vi "AMZ_S3_APIHLP_Convert MFA Delete String to Enum.vi"(4 "MFA Delete String":string) -> (1 "MFA Delete":T1)   [LabVIEW 2015, in "LV Interface for Amazon S3.lvlib"]
doc: "Convert the Storage Class represented as a String to the Enum typedef representation."
uses:
  LV Interface for Amazon S3.lvlib
  Typedefs/AMZ_S3_MFA Delete.ctl
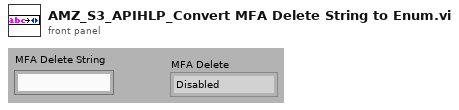
[diagram p1: front panel]
types:
  T1 = typedef "LV Interface for Amazon S3.lvlib/AMZ_S3_MFA Delete.ctl" = enum16{"Disabled", "Enabled"}
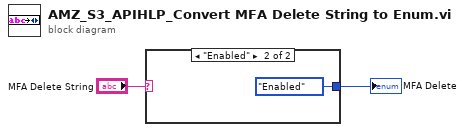
[diagram p0: block diagram]
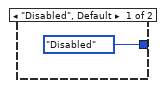
[diagram p2: hidden frame]
diagram:
  n1 = case shown="\"Enabled\"" "MFA Delete String" {
    tunnel: [AMZ_S3_MFA_Delete."Disabled" ("MFA Delete") AMZ_S3_MFA_Delete."Enabled" ("MFA Delete")] -> w1
    frame "Disabled", Default {
    }
    frame "Enabled" {
    }
  }
  "MFA Delete" <- w1
